vi "Correct_Choice_of_Basis_Subtrack-1.vi"(4 "error IN":errorcluster, 5 "[IN] # of Longest track\nInside the Group of Tracks":i32, 6 "[IN] Index of Earliest \nProblem Point Inside":i32, 7 "[IN] Still connected\ntracks in group":T1) -> (0 "error OUT":errorcluster, 1 "[OUT] # of Correc\nted Longest Track":i32, 2 "[OUT] # of Prob\nlem Point Inside":i32)   [LabVIEW 2013]
doc: "SubVI corrects the case of \"101\" (merging) point connected with \"111\" (splitting) because SPLITTING point should be resolved first (!) before merging event resolving"
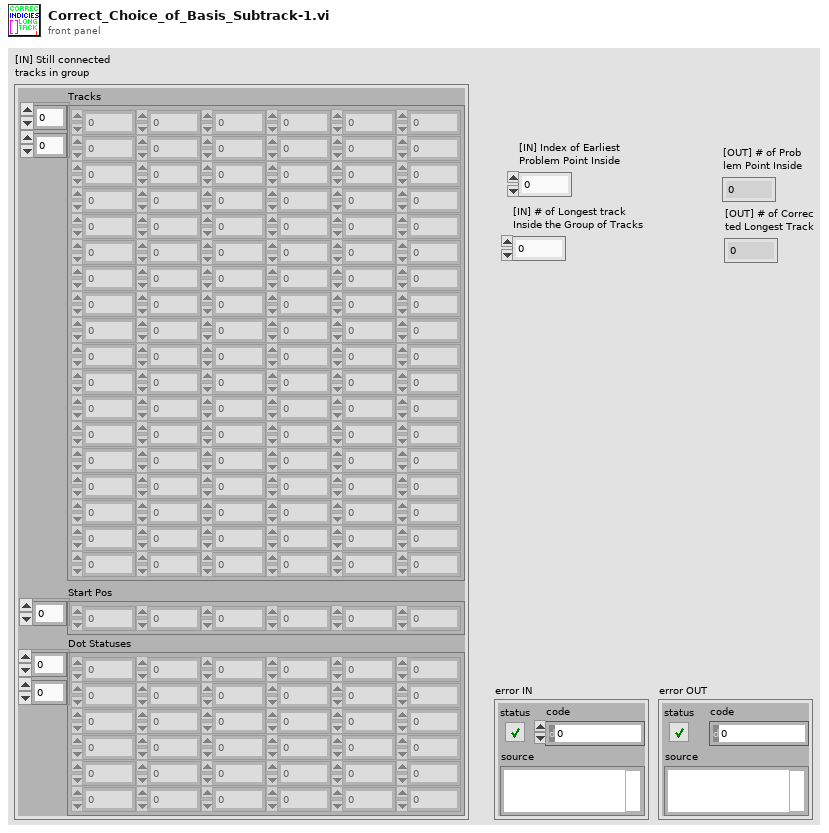
[diagram p1: front panel]
types:
  T1 = cluster{"Tracks":dbl[][], "Start Pos":i32[], "Dot Statuses":i16[][]}
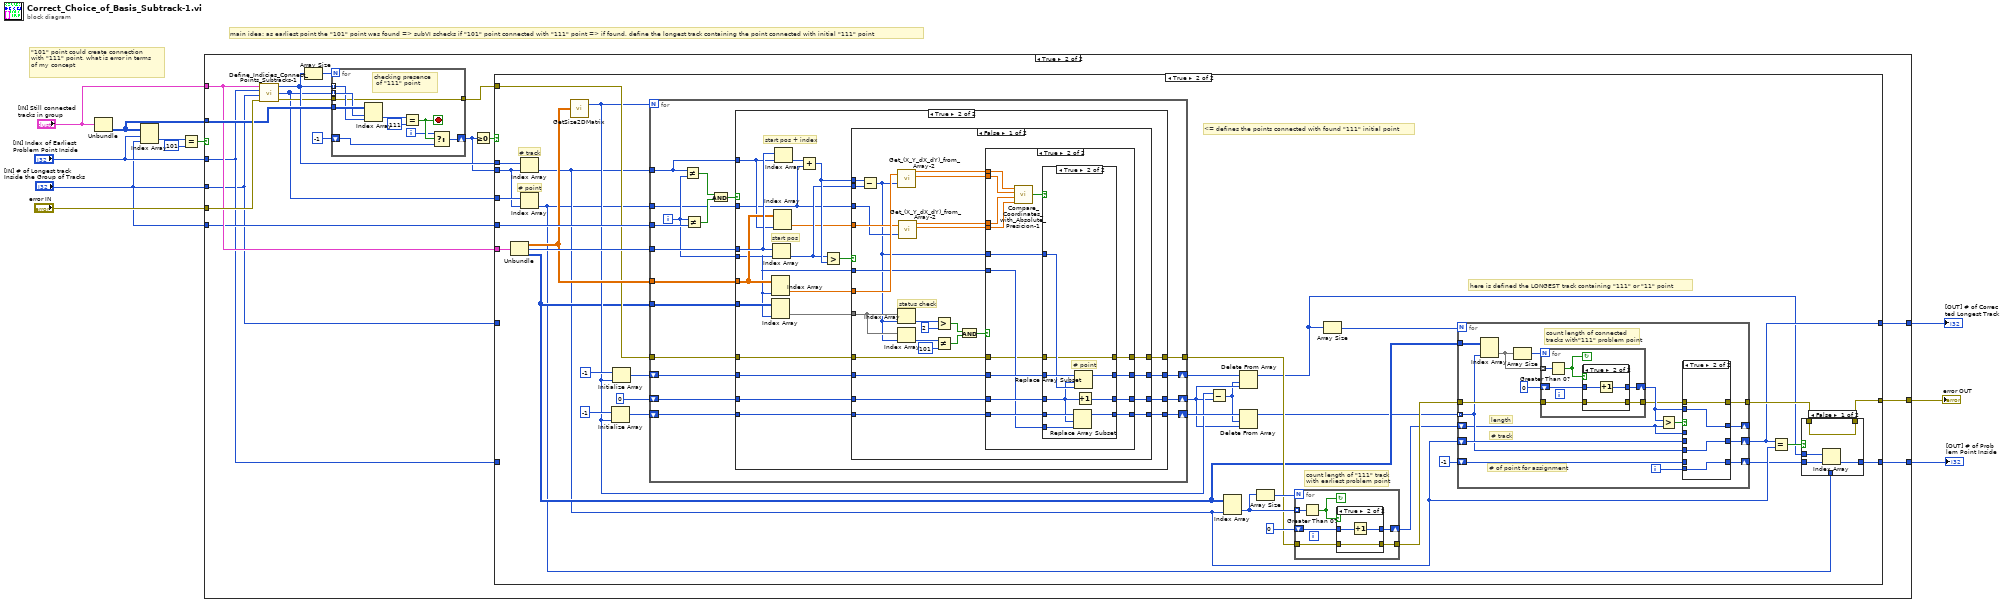
[diagram p0: block diagram]
diagram:
  # "main idea: as earliest point the \"101\" point was found => subVI schecks if \"101\" point connected with \"111\" point => if found, define the longest track containing the point connected with initial \"111\" point"
  # "\"101\" point could create connection \nwith \"111\" point, what is error in terms \nof my concept"
  n1 = Unbundle("[IN] Still connected\ntracks in group") -> ("Dot Statuses"=w5:i16[][])  [unwired: 2 out]
  n2 = Index Array(array=w5, index (row)="[IN] Index of Earliest \nProblem Point Inside", index (col)="[IN] # of Longest track\nInside the Group of Tracks") -> (element=w11:i16)
  n3 = Equal?(x=w11, y=i16 101) -> (x = y?=w9:bool)
  n4 = case shown="True" w9 {
    tunnel: "error IN" -> [w13 w31]
    tunnel: "[IN] Still connected\ntracks in group" -> [_ w21]
    tunnel: "[IN] Index of Earliest \nProblem Point Inside" -> [w12 w16]
    tunnel: "[IN] # of Longest track\nInside the Group of Tracks" -> [_ w15]
    tunnel: w5 -> [_ w29]
    tunnel: "[IN] # of Longest track\nInside the Group of Tracks" -> [w14 w20]
    tunnel: [w12 w19] -> w1
    tunnel: [w13 w18] -> w2
    tunnel: [w14 w17] -> w3
    frame False {
    }
    frame True {
      n5 = call "Define_Indicies_Connect_Points_Subtracks-1.vi"("error IN"=w31, "[IN] Index of track with\n(problem displacement)"=w15, "[IN] Index of problem\ndisplacement inside track"=w16, "[IN] Track group"=w21) -> ("error OUT"=w25:errorcluster, "[OUT] Index of \nconnected dots\ninside the track"=w24:i32[], "[OUT] Index of connected\ntracks with problem dot"=w26:i32[])
      n6 = Array Size(array=w26) -> (size(s)=w30:i32)
      n7 = for {
        N: w30 -> [_]
        tunnel: w26 -> [w238] mode=indexing
        tunnel: w24 -> [w239] mode=indexing
        tunnel: w29 -> [w240]
        shift-right: [w233] -> w23
        shift-left: -1 -> [w234]
        tunnel: w25 -> [w231]
        tunnel: [w231] -> w22
        i -> [w232]
        stop <- w235 stop-if-true
        # "checking presence\n of \"111\" point"
        n8 = Index Array(array=w240, index (row)=w239, index (col)=w238) -> (element=w236:i16)
        n9 = Equal?(x=w236, y=i16 111) -> (x = y?=w235:bool)
        n10 = Select(t=w232, s=w235, f=w234) -> (s? t:f=w233:i32)
      }
      n11 = Greater Or Equal To 0?(x=w23) -> (x >= 0?=w27:bool)
      n12 = case shown="True" w27 {
        tunnel: w26 -> [_ w71]
        tunnel: w24 -> [_ w70]
        tunnel: w23 -> [_ w69]
        tunnel: w22 -> [w34 w59]
        tunnel: w21 -> [_ w68]
        tunnel: w20 -> [_ w66]
        tunnel: [w32 w40] -> w17
        tunnel: [w34 w37] -> w18
        tunnel: [w33 w36] -> w19
        tunnel: w16 -> [w33 _]
        tunnel: w15 -> [w32 _]
        frame False {
        }
        frame True {
          # "here is defined the LONGEST track containing \"111\" or \"11\" point"
          # "<= defines the points connected with found \"111\" initial point"
          # "count length of \"111\" track\nwith earliest problem point"
          # "# point"
          # "# track"
          n13 = Unbundle(w68) -> ("Tracks"=w62:dbl[][], "Start Pos"=w67:i32[], "Dot Statuses"=w48:i16[][])
          n14 = Index Array(array=w71, index=w69) -> (element=w44:i32)
          n15 = Index Array(array=w70, index=w69) -> (element=w38:i32)
          n16 = call "GetSize2DMatrix.vi"("Array IN (2D)"=w62) -> ("# Cols"=w56:i32)  [unwired: 1 out]
          n17 = Initialize Array(-1, w56) -> (w60:i32[])
          n18 = Initialize Array(-1, w56) -> (w61:i32[])
          n19 = for {
            N: w56 -> [_]
            tunnel: w67 -> [w138]
            tunnel: w44 -> [w136]
            tunnel: w38 -> [w135]
            tunnel: w66 -> [w142]
            shift-right: [w128] -> w55
            shift-left: 0 -> [w130]
            tunnel: w62 -> [w134]
            tunnel: w48 -> [w133]
            shift-right: [w129] -> w58
            shift-left: w61 -> [w131]
            shift-right: [w126] -> w57
            shift-left: w60 -> [w127]
            tunnel: w59 -> [w132]
            tunnel: [w125] -> w50
            i -> [w137]
            n20 = Not Equal?(x=w136, y=w137) -> (x != y?=w140:bool)
            n21 = Not Equal?(x=w137, y=w142) -> (x != y?=w141:bool)
            n22 = And(x=w140, y=w141) -> (x .and. y?=w139:bool)
            n23 = case shown="True" w139 {
              tunnel: w138 -> [_ w167]
              tunnel: w137 -> [_ w153]
              tunnel: w136 -> [_ w158]
              tunnel: w135 -> [_ w156]
              tunnel: w134 -> [_ w159]
              tunnel: w133 -> [_ w161]
              tunnel: w132 -> [w143 w155]
              tunnel: w131 -> [w146 w154]
              tunnel: w130 -> [w145 w152]
              tunnel: [w146 w151] -> w129
              tunnel: [w145 w150] -> w128
              tunnel: w127 -> [w144 w149]
              tunnel: [w144 w148] -> w126
              tunnel: [w143 w147] -> w125
              frame False {
              }
              frame True {
                # "start pos"
                # "start pos + index"
                n24 = Index Array(array=w159, index (col)=w153) -> (element=w162:dbl[])  [unwired: 1 in]
                n25 = Index Array(array=w161, index (col)=w153) -> (element=w160:i16[])  [unwired: 1 in]
                n26 = Index Array(array=w167, index=w153) -> (element=w163:i32)
                n27 = Index Array(array=w159, index (col)=w158) -> (element=w157:dbl[])  [unwired: 1 in]
                n28 = Index Array(array=w167, index=w158) -> (element=w166:i32)
                n29 = Add(x=w166, y=w156) -> (x+y=w164:i32)
                n30 = Greater?(x=w163, y=w164) -> (0:w165:bool)
                n31 = case shown="False" w165 {
                  tunnel: w164 -> [w194 _]
                  tunnel: w163 -> [w193 _]
                  tunnel: w162 -> [w192 _]
                  tunnel: w160 -> [w189 _]
                  tunnel: w157 -> [w183 _]
                  tunnel: w156 -> [w182 _]
                  tunnel: w155 -> [w177 w227]
                  tunnel: w154 -> [w176 w230]
                  tunnel: w153 -> [w175 _]
                  tunnel: w152 -> [w173 w229]
                  tunnel: [w172 w230] -> w151
                  tunnel: [w171 w229] -> w150
                  tunnel: w149 -> [w170 w228]
                  tunnel: [w169 w228] -> w148
                  tunnel: [w168 w227] -> w147
                  frame False {
                    # "status check"
                    n32 = Subtract(x=w194, y=w193) -> (x-y=w174:i32)
                    n33 = Index Array(array=w189, index=w174) -> (element=w188:i16)
                    n34 = call "Get_(X_Y_dX_dY)_from_Array-2.vi"("(X,Y,dX,dY)"=w192, "Index of Displacement"=w174) -> ("X"=w181:dbl, "Y"=w180:dbl)  [unwired: 2 out]
                    n35 = Index Array(array=w189, index=w174) -> (element=w191:i16)
                    n36 = call "Get_(X_Y_dX_dY)_from_Array-2.vi"("(X,Y,dX,dY)"=w183, "Index of Displacement"=w182) -> ("X"=w179:dbl, "Y"=w178:dbl)  [unwired: 2 out]
                    n37 = Greater?(x=w191, y=i16 2) -> (0:w186:bool)
                    n38 = Not Equal?(x=w188, y=i16 101) -> (x != y?=w185:bool)
                    n39 = And(x=w186, y=w185) -> (x .and. y?=w184:bool)
                    n40 = case shown="True" w184 {
                      tunnel: w181 -> [_ w213]
                      tunnel: w180 -> [_ w212]
                      tunnel: w179 -> [_ w211]
                      tunnel: w178 -> [_ w210]
                      tunnel: w177 -> [w195 w200]
                      tunnel: w176 -> [w198 w208]
                      tunnel: w175 -> [_ w202]
                      tunnel: w174 -> [_ w207]
                      tunnel: w173 -> [w197 w206]
                      tunnel: [w198 w205] -> w172
                      tunnel: [w197 w204] -> w171
                      tunnel: w170 -> [w196 w203]
                      tunnel: [w196 w201] -> w169
                      tunnel: [w195 w199] -> w168
                      frame False {
                      }
                      frame True {
                        n41 = call "Compare_Coordinates_with_Absolute_Presicion-1.vi"("X 1"=w213, "Y 1"=w212, "X 2"=w211, "Y 2"=w210) -> ("[OUT] Same coordinates?"=w209:bool)  [unwired: 1 in]
                        n42 = case shown="True" w209 {
                          tunnel: w208 -> [w217 w226]
                          tunnel: w207 -> [_ w225]
                          tunnel: w206 -> [w216 w221]
                          tunnel: [w217 w224] -> w205
                          tunnel: [w216 w223] -> w204
                          tunnel: w203 -> [w215 w222]
                          tunnel: w202 -> [_ w220]
                          tunnel: [w215 w219] -> w201
                          tunnel: w200 -> [w214 w218]
                          tunnel: [w214 w218] -> w199
                          frame False {
                          }
                          frame True {
                            # "# point"
                            n43 = Replace Array Subset(array=w222, new element=w220, index=w221) -> (w219:i32[])
                            n44 = Replace Array Subset(array=w226, new element=w225, index=w221) -> (w224:i32[])
                            n45 = Increment(x=w221) -> (x+1=w223:i32)
                          }
                        }
                      }
                    }
                  }
                  frame True {
                  }
                }
              }
            }
          }
          n46 = Subtract(x=w56, y=w55) -> (x-y=w54:i32)
          n47 = Index Array(array=w48, index (col)=w44) -> (element=w52:i16[])  [unwired: 1 in]
          n48 = Delete From Array(array=w57, length=w54, index=w55) -> (array with subset deleted=w41:i32[])  [unwired: 1 out]
          n49 = Delete From Array(array=w58, length=w54, index=w55) -> (array with subset deleted=w35:i32[])  [unwired: 1 out]
          n50 = Array Size(array=w52) -> (size(s)=w53:i32)
          n51 = for {
            N: w53 -> [_]
            tunnel: w52 -> [w119] mode=indexing
            shift-right: [w116] -> w46
            shift-left: 0 -> [w117]
            tunnel: w50 -> [w115]
            tunnel: [w114] -> w47
            stop <- w118 continue-if-true
            n52 = Greater Than 0?(x=w119) -> (x > 0?=w118:bool)
            n53 = case shown="True" w118 {
              tunnel: w117 -> [w121 w124]
              tunnel: [w121 w123] -> w116
              tunnel: w115 -> [w120 w122]
              tunnel: [w120 w122] -> w114
              frame False {
              }
              frame True {
                n54 = Increment(x=w124) -> (x+1=w123:i32)
              }
            }
          }
          n55 = Array Size(array=w35) -> (size(s)=w49:i32)
          n56 = for {
            N: w49 -> [_]
            tunnel: w41 -> [w85] mode=indexing
            tunnel: w48 -> [w94]
            tunnel: w47 -> [w90]
            shift-right: [w87] -> _
            shift-left: w46 -> [w83]
            shift-right: [w84] -> w40
            shift-left: w44 -> [w86]
            shift-right: [w80] -> w39
            shift-left: -1 -> [w82]
            tunnel: [w78] -> w42
            i -> [w81]
            # "# of point for assignment"
            # "# track"
            # "length"
            # "count length of connected \ntracks with\"111\" problem point"
            n57 = Index Array(array=w94, index (col)=w85) -> (element=w91:i16[])  [unwired: 1 in]
            n58 = Array Size(array=w91) -> (size(s)=w93:i32)
            n59 = for {
              N: w93 -> [_]
              tunnel: w91 -> [w108] mode=indexing
              shift-right: [w105] -> w88
              shift-left: 0 -> [w106]
              tunnel: w90 -> [w104]
              tunnel: [w103] -> w79
              stop <- w107 continue-if-true
              n60 = Greater Than 0?(x=w108) -> (x > 0?=w107:bool)
              n61 = case shown="True" w107 {
                tunnel: w106 -> [w110 w113]
                tunnel: [w110 w112] -> w105
                tunnel: w104 -> [w109 w111]
                tunnel: [w109 w111] -> w103
                frame False {
                }
                frame True {
                  n62 = Increment(x=w113) -> (x+1=w112:i32)
                }
              }
            }
            n63 = Greater?(x=w88, y=w83) -> (0:w89:bool)
            n64 = case shown="True" w89 {
              tunnel: w88 -> [_ w102]
              tunnel: [w97 w102] -> w87
              tunnel: w86 -> [w98 _]
              tunnel: w85 -> [_ w101]
              tunnel: [w98 w101] -> w84
              tunnel: w83 -> [w97 _]
              tunnel: w82 -> [w96 _]
              tunnel: w81 -> [_ w100]
              tunnel: [w96 w100] -> w80
              tunnel: w79 -> [w95 w99]
              tunnel: [w95 w99] -> w78
              frame False {
              }
              frame True {
              }
            }
          }
          n65 = Equal?(x=w40, y=w44) -> (x = y?=w43:bool)
          n66 = case shown="False" w43 {
            tunnel: w42 -> [w75 w77]
            tunnel: [w75 w77] -> w37
            tunnel: w35 -> [w74 _]
            tunnel: [w72 w76] -> w36
            tunnel: w39 -> [w73 _]
            tunnel: w38 -> [_ w76]
            frame False {
              n67 = Index Array(array=w74, index=w73) -> (element=w72:i32)
            }
            frame True {
            }
          }
        }
      }
    }
  }
  "error OUT" <- w2
  "[OUT] # of Correc\nted Longest Track" <- w3
  "[OUT] # of Prob\nlem Point Inside" <- w1
